vi "Alarm.vi"(11 "Menu Ring":u16(ring) items=["Amber", "OMFG"]) -> ()   [LabVIEW 2017]
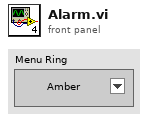
[diagram p1: front panel]
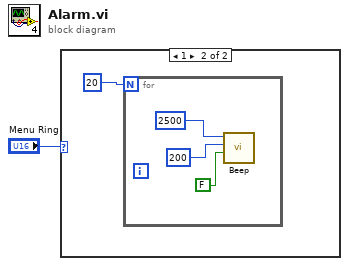
[diagram p0: block diagram]
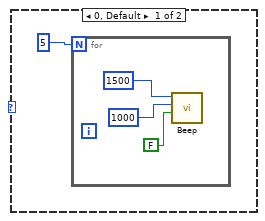
[diagram p2: hidden frame]
diagram:
  n1 = case shown="1" "Menu Ring" {
    frame 0, Default {
      n2 = for {
        N: 5 -> [_]
        n3 = call <vilib>:"Beep.vi"("use system alert? (T)"=FALSE, "duration (msec)"=u32 1000, "frequency (Hz)"=u32 1500) -> ()  [unwired: 9 in]
      }
    }
    frame 1 {
      n4 = for {
        N: 20 -> [_]
        n5 = call <vilib>:"Beep.vi"("use system alert? (T)"=FALSE, "duration (msec)"=u32 200, "frequency (Hz)"=u32 2500) -> ()  [unwired: 9 in]
      }
    }
  }
